vi "T7MOD_Read_FLOAT32_Registers.vi"(6 "Num Reg":i32=2, 8 "error in":errorcluster, 9 "Starting FLOAT32 Register":i32=55124, 10 "Remote Port":u16=502, 11 "Remote IP Address":string="192.168.1.15") -> (0 "error out":errorcluster, 1 "Read At":timestamp, 2 "Raw Data Read":u16[](array[numeric]), 3 "Read FLOAT32":sgl[](array[numeric]))   [LabVIEW 2018]
panel:
  # "Output"
  # "TCP Parameters"
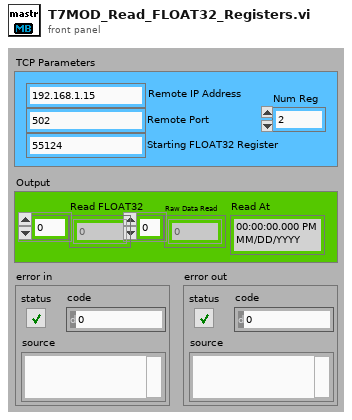
[diagram p1: front panel]
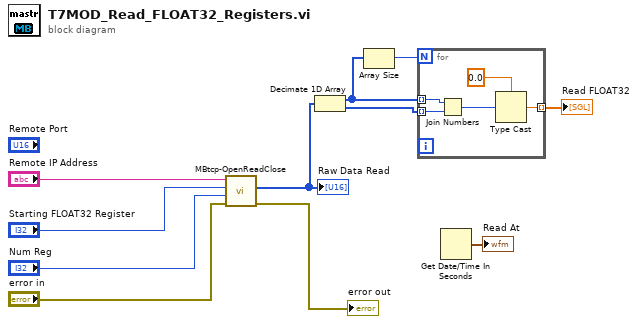
[diagram p0: block diagram]
diagram:
  n1 = call "MBtcp-OpenReadClose.vi"("error in (no error)"="error in", "nRegisters"="Num Reg", "RegisterAddr"="Starting FLOAT32 Register", "IP Address(:port)"="Remote IP Address") -> ("error out"=→"error out":errorcluster, "16bitValues"=w1:u16[])  [unwired: 5 in, 1 out]
  "Raw Data Read" <- w1
  n2 = Decimate 1D Array(w1) -> (w8:u16[], w11:u16[])
  n3 = Array Size(array=w8) -> (size(s)=w7:i32)
  n4 = for {
    N: w7 -> [_]
    tunnel: w8 -> [w16] mode=indexing
    tunnel: w11 -> [w15] mode=indexing
    tunnel: [w12] -> w10 mode=indexing
    n5 = Join Numbers(hi=w16, lo=w15) -> ((hi.lo)=w14:u32)
    n6 = Type Cast(type=sgl 0.0 ("type: FLOAT32"), x=w14) -> (*(type *) &x=w12:sgl)
  }
  "Read FLOAT32" <- w10
  n7 = Get Date/Time In Seconds() -> (seconds since 1Jan1904=→"Read At":timestamp)
